vi "to_json.vi"(8 "error in":errorcluster, 11 "ts.absoloute in":refnum<class "ts.absoloute.lvclass">) -> (0 "error out":errorcluster, 2 "json":string, 3 "ts.absoloute out":refnum<class "ts.absoloute.lvclass">, 4 "Not Default":bool)   [LabVIEW 2020, in "ts.absoloute.lvclass"]
uses:
  ts.absoloute.lvclass
  ts.absoloute.lvclass/ts.absoloute.ctl
  <vilib>/JDP Science/JSONtext/support/Format JSON Object.vi
  ts.absoloute type/ts.absoloute type.lvclass
  <vilib>/JDP Science/JSONtext/JSONtext.lvlib
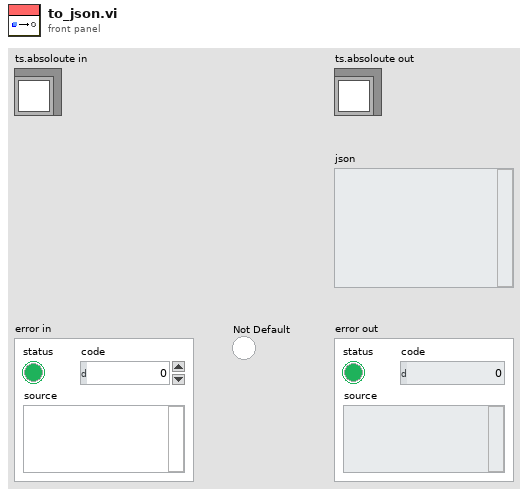
[diagram p1: front panel]
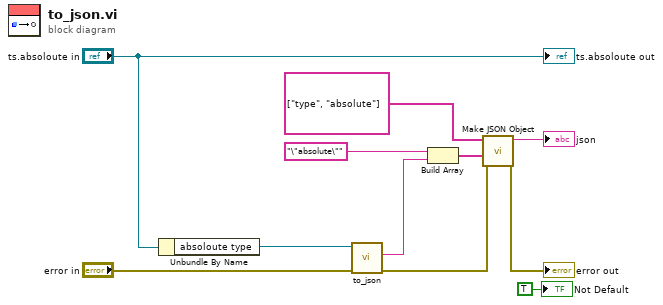
[diagram p0: block diagram]
diagram:
  n1 = Unbundle By Name("ts.absoloute in") -> ("absoloute type"=w3:refnum<class "ts.absoloute type.lvclass">)
  n2 = call-dynamic "to_json.vi"("error in"="error in", "ts.absoloute type in"=w3) -> ("error out"=w5:errorcluster, "json"=w6:string)  [unwired: 6 in, 2 out]
  n3 = Build Array("\"absolute\"" ("String"), w6) -> (w7:string[])
  n4 = call <vilib>:"Make JSON Object.vi"("error in (no error)"=w5, "JSON Items"=w7, "Item Names"=string[] ["type", "absolute"]) -> ("error out"=→"error out":errorcluster, "<JSON>"=→"json":string)  [unwired: 7 in]
  "ts.absoloute out" <- "ts.absoloute in"
  "Not Default" <- TRUE ("Not Default")
